vi "Parse Single Item.vi"(7 "Quoted String? (F)":bool, 11 "String In":string) -> (2 "Remaining":string, 3 "Item":string, 5 "JSON Item Type":T1=enum."null")   [LabVIEW 2020, in "JSON.lvlib"]
doc: "Separates out and determines the type of the next value in the string input. This is typically used after a property name string has been removed and then the value and type need to be pulled out for that property key."
uses:
  JSON.lvlib
  <vilib>/regexp/Match Regular Expression.xnode
  JSON Item Type.ctl
  <vilib>/Utility/error.llb/whitespace.ctl
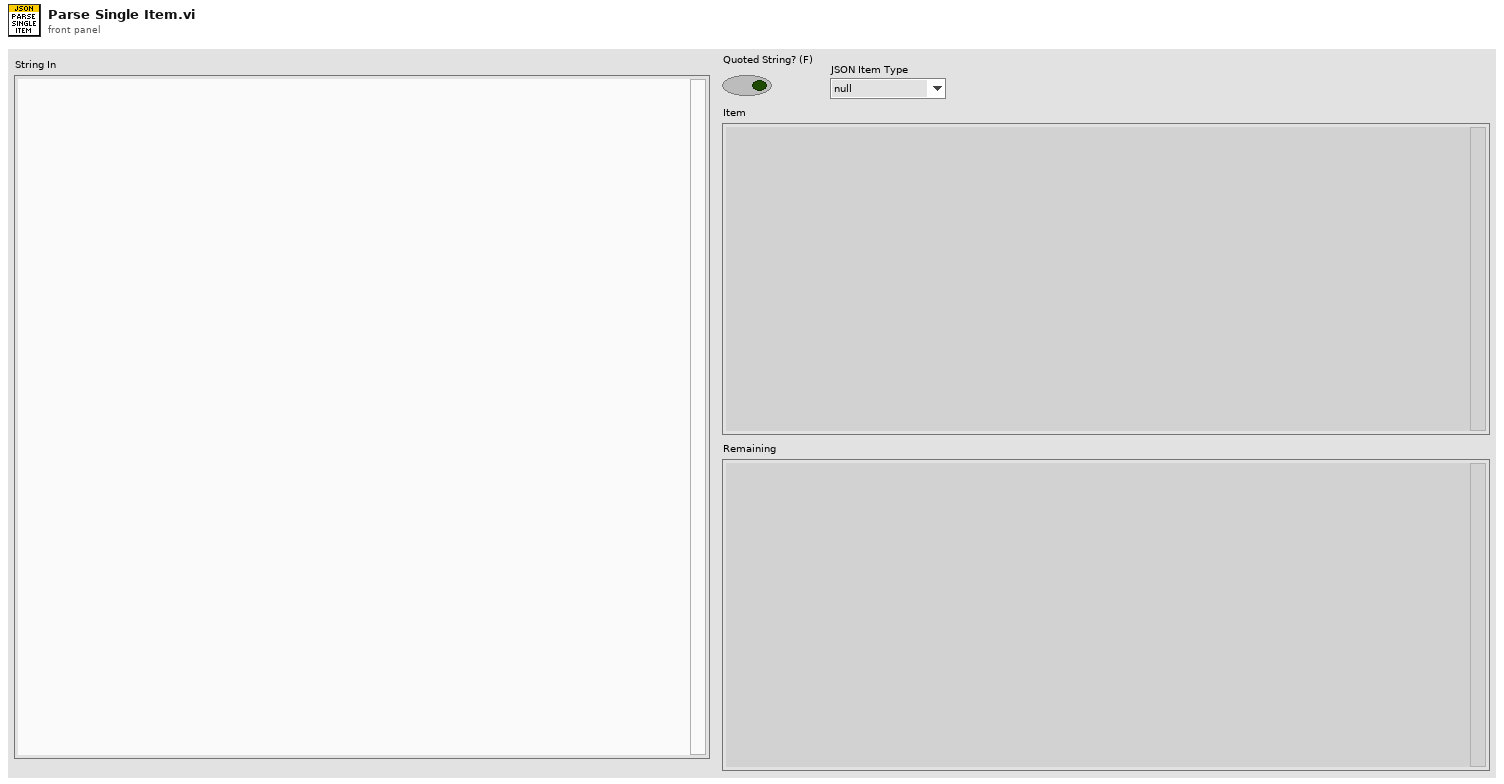
[diagram p1: front panel]
types:
  T1 = typedef "JSON.lvlib/JSON Item Type.ctl" = enum16{"unknown", "null", "Array", "Object", "String", "Number", "Boolean"}
  T2 = typedef "whitespace.ctl" = u16
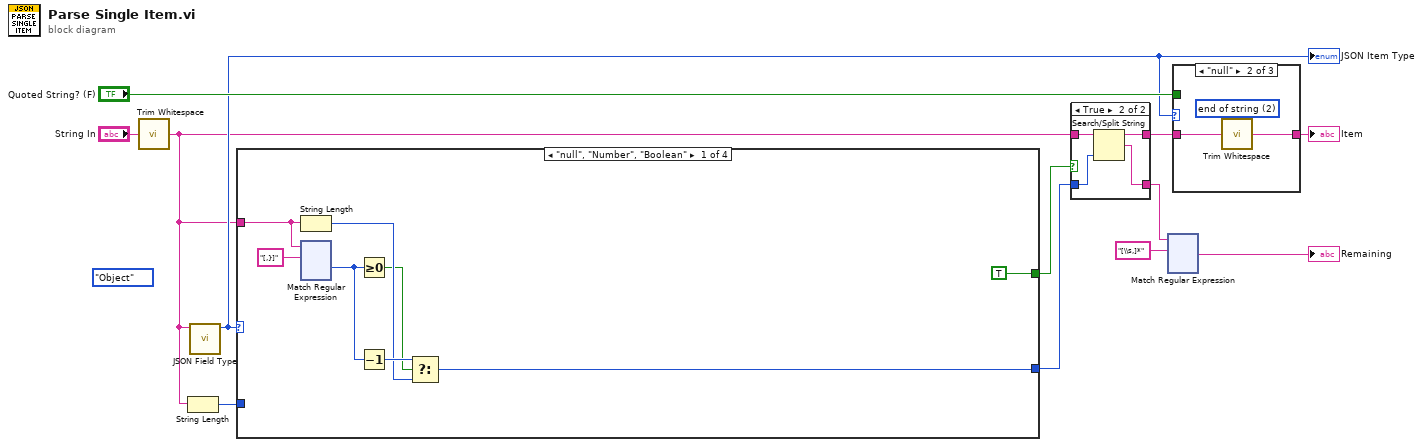
[diagram p0: block diagram]
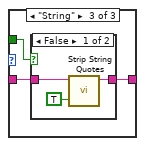
[diagram p3: hidden frame]
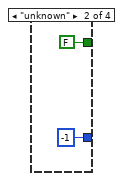
[diagram p5: hidden frame]
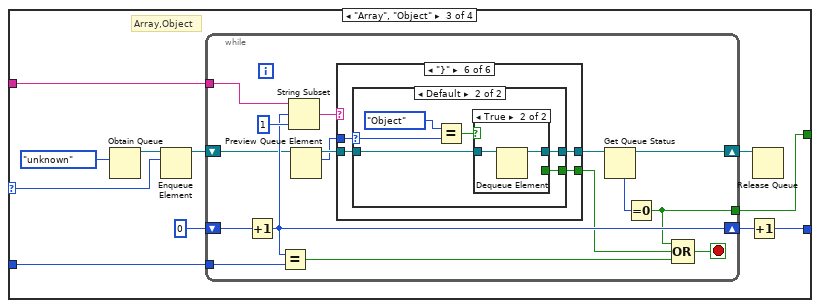
[diagram p6: hidden frame]
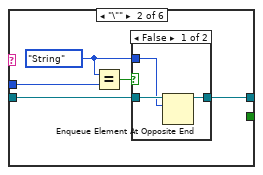
[diagram p8: hidden frame]
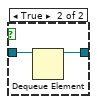
[diagram p9: hidden frame]
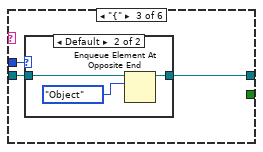
[diagram p10: hidden frame]
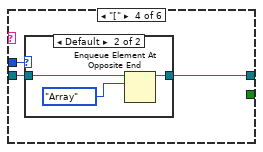
[diagram p12: hidden frame]
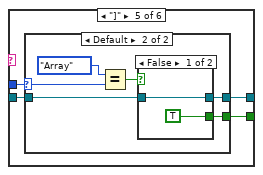
[diagram p14: hidden frame]
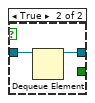
[diagram p16: hidden frame]
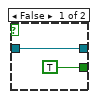
[diagram p18: hidden frame]
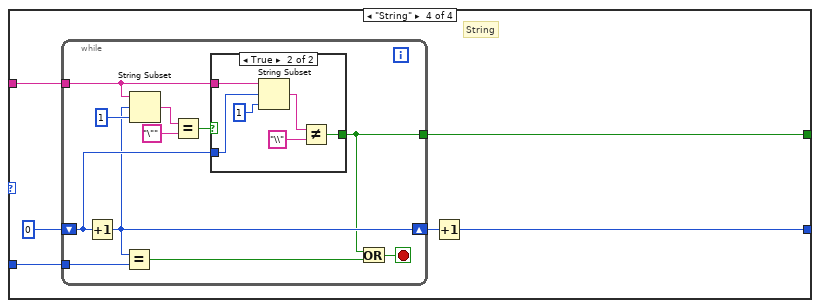
[diagram p19: hidden frame]
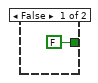
[diagram p20: hidden frame]
diagram:
  (unwired) JSON_Item_Type."Object" ("JSON Item Type")
  n1 = call <vilib>:"Trim Whitespace.vi"("string"="String In") -> ("trimmed string"=w1:string)  [unwired: 1 in]
  n2 = String Length(string=w1) -> (length=w11:i32)
  n3 = call "JSON Field Type.vi"("JSON String"=w1) -> ("JSON Item Type"=w2:T1)  [unwired: 10 in]
  "JSON Item Type" <- w2
  n4 = case shown="\"null\", \"Number\", \"Boolean\"" w2 {
    selector: w2 -> [_ _ w149 _]
    tunnel: w1 -> [w18 _ w147 w227]
    tunnel: w11 -> [_ _ w145 w226]
    tunnel: [w13 -1 w142 w222] -> w10
    tunnel: [TRUE FALSE w144 w223] -> w9
    frame "null", "Number", "Boolean" {
      n5 = String Length(string=w18) -> (length=w16:i32)
      n6 = xnode "Match Regular Expression"("input string"=w18, "regular expression"="[,}]") -> ("offset past match"=w19:i32)  [unwired: 4 in, 4 out]
      n7 = Greater Or Equal To 0?(x=w19) -> (x >= 0?=w15:bool)
      n8 = Decrement(x=w19) -> (x-1=w17:i32)
      n9 = Select(t=w17, s=w15, f=w16) -> (s? t:f=w13:i32)
    }
    frame "unknown" {
    }
    frame "Array", "Object" {
      # "Array,Object"
      n10 = Obtain Queue(element data type=JSON_Item_Type."unknown" ("JSON Item Type")) -> (queue out=w150:refnum<queue>)  [unwired: 4 in, 2 out]
      n11 = Enqueue Element(queue=w150, element=w149) -> (queue out=w148:refnum<queue>)  [unwired: 2 in, 2 out]
      n12 = while {
        shift-right: [w153] -> w141
        shift-left: w148 -> [w158]
        tunnel: w147 -> [w163]
        shift-right: [w159] -> w143
        shift-left: 0 -> [w161]
        tunnel: w145 -> [w166]
        tunnel: [w151] -> w144
        stop <- w164 stop-if-true
        n13 = Increment(x=w161) -> (x+1=w159:i32)
        n14 = Equal?(x=w159, y=w166) -> (x = y?=w165:bool)
        n15 = String Subset(string=w163, offset (0)=w159, length (rest)=1 ("length (rest)")) -> (substring=w160:string)
        n16 = Preview Queue Element(queue=w158) -> (queue out=w157:refnum<queue>, element=w156:T1)  [unwired: 2 in, 2 out]
        n17 = case shown="\"}\"" w160 {
          tunnel: w156 -> [_ w171 w178 w185 w193 w208]
          tunnel: w157 -> [w167 w170 w180 w187 w195 w210]
          tunnel: [w167 w169 w179 w186 w194 w209] -> w154
          tunnel: [_ _ _ _ w192 w207] -> w155
          frame Default {
          }
          frame "\"" {
            w168 = JSON_Item_Type."String" ("JSON Item Type")
            n18 = Equal?(x=w168, y=w171) -> (x = y?=w172:bool)
            n19 = case shown="False" w172 {
              tunnel: w170 -> [w175 w177]
              tunnel: [w174 w176] -> w169
              tunnel: w168 -> [w173 _]
              frame False {
                n20 = Enqueue Element At Opposite End(queue=w175, element=w173) -> (queue out=w174:refnum<queue>)  [unwired: 2 in, 2 out]
              }
              frame True {
                n21 = Dequeue Element(queue=w177) -> (queue out=w176:refnum<queue>)  [unwired: 2 in, 3 out]
              }
            }
          }
          frame "{" {
            n22 = case shown="Default" w178 {
              tunnel: w180 -> [w181 w184]
              tunnel: [w181 w183] -> w179
              frame "String" {
              }
              frame Default {
                n23 = Enqueue Element At Opposite End(queue=w184, element=JSON_Item_Type."Object" ("JSON Item Type")) -> (queue out=w183:refnum<queue>)  [unwired: 2 in, 2 out]
              }
            }
          }
          frame "[" {
            n24 = case shown="Default" w185 {
              tunnel: w187 -> [w188 w191]
              tunnel: [w188 w190] -> w186
              frame "String" {
              }
              frame Default {
                n25 = Enqueue Element At Opposite End(queue=w191, element=JSON_Item_Type."Array" ("JSON Item Type")) -> (queue out=w190:refnum<queue>)  [unwired: 2 in, 2 out]
              }
            }
          }
          frame "]" {
            n26 = case shown="Default" w193 {
              selector: w193 -> [_ w202]
              tunnel: w195 -> [w196 w200]
              tunnel: [w196 w199] -> w194
              tunnel: [_ w198] -> w192
              frame "String" {
              }
              frame Default {
                n27 = Equal?(x=JSON_Item_Type."Array" ("JSON Item Type"), y=w202) -> (x = y?=w201:bool)
                n28 = case shown="False" w201 {
                  tunnel: w200 -> [w204 w206]
                  tunnel: [w204 w205] -> w199
                  tunnel: [TRUE _] -> w198
                  frame False {
                  }
                  frame True {
                    n29 = Dequeue Element(queue=w206) -> (queue out=w205:refnum<queue>)  [unwired: 2 in, 3 out]
                  }
                }
              }
            }
          }
          frame "}" {
            n30 = case shown="Default" w208 {
              selector: w208 -> [_ w217]
              tunnel: w210 -> [w211 w215]
              tunnel: [w211 w214] -> w209
              tunnel: [_ w213] -> w207
              frame "String" {
              }
              frame Default {
                n31 = Equal?(x=JSON_Item_Type."Object" ("JSON Item Type"), y=w217) -> (x = y?=w216:bool)
                n32 = case shown="True" w216 {
                  tunnel: w215 -> [w219 w221]
                  tunnel: [w219 w220] -> w214
                  tunnel: [TRUE _] -> w213
                  frame False {
                  }
                  frame True {
                    n33 = Dequeue Element(queue=w221) -> (queue out=w220:refnum<queue>)  [unwired: 2 in, 3 out]
                  }
                }
              }
            }
          }
        }
        n34 = Get Queue Status(queue=w154) -> (queue out=w153:refnum<queue>, # elements in queue=w152:i32)  [unwired: 2 in, 6 out]
        n35 = Equal To 0?(x=w152) -> (x = 0?=w151:bool)
        n36 = Compound Arithmetic op=OR(w151, w155, w165) -> (w164:bool)
      }
      n37 = Increment(x=w143) -> (x+1=w142:i32)
      n38 = Release Queue(queue=w141) -> ()  [unwired: 2 in, 3 out]
    }
    frame "String" {
      # "String"
      n39 = while {
        tunnel: w227 -> [w232]
        shift-right: [w230] -> w224
        shift-left: 0 ("length (rest)") -> [w231]
        tunnel: w226 -> [w238]
        tunnel: [w229] -> w223
        stop <- w237 stop-if-true
        n40 = Increment(x=w231) -> (x+1=w230:i32)
        n41 = Equal?(x=w230, y=w238) -> (x = y?=w236:bool)
        n42 = String Subset(string=w232, offset (0)=w230, length (rest)=1 ("length (rest)")) -> (substring=w234:string)
        n43 = Equal?(x=w234, y="\"") -> (x = y?=w233:bool)
        n44 = case shown="True" w233 {
          tunnel: w232 -> [_ w244]
          tunnel: w231 -> [_ w243]
          tunnel: [FALSE w240] -> w229
          frame False {
          }
          frame True {
            n45 = String Subset(string=w244, offset (0)=w243, length (rest)=1 ("length (rest)")) -> (substring=w242:string)
            n46 = Not Equal?(x=w242, y="\\") -> (x != y?=w240:bool)
          }
        }
        n47 = Or(x=w229, y=w236) -> (x .or. y?=w237:bool)
      }
      n48 = Increment(x=w224) -> (x+1=w222:i32)
    }
  }
  n49 = case shown="True" w9 {
    tunnel: w1 -> [w247 w251]
    tunnel: w10 -> [_ w250]
    tunnel: ["" ("trimmed string") w249] -> w5
    tunnel: [w247 w248] -> w8
    frame False {
    }
    frame True {
      n50 = Search/Split String(string=w251, offset (0)=w250) -> (substring before match=w249:string, match + rest of string=w248:string)  [unwired: 1 in, 1 out]
    }
  }
  n51 = xnode "Match Regular Expression"("input string"=w8, "regular expression"="[\\s,]*") -> ("after match"=→"Remaining":string)  [unwired: 4 in, 4 out]
  n52 = case shown="\"null\"" w2 {
    tunnel: w5 -> [w252 w255 w258]
    tunnel: [w252 w254 w257] -> w4
    tunnel: "Quoted String? (F)" -> [_ _ w256]
    frame Default {
    }
    frame "null" {
      w253 = T2 2 items=["both", "start of string", "end of string"] ("location (both)")
      n53 = call <vilib>:"Trim Whitespace.vi"("string"=w255, "location (both)"=w253) -> ("trimmed string"=w254:string)
    }
    frame "String" {
      n54 = case shown="False" w256 {
        tunnel: w258 -> [w261 w262]
        tunnel: [w259 w262] -> w257
        frame False {
          n55 = call "Strip String Quotes.vi"("Skip Type Check? (F)"=TRUE, "JSON"=w261) -> ("Quotes Stripped"=w259:string)  [unwired: 9 in]
        }
        frame True {
        }
      }
    }
  }
  "Item" <- w4
